vi "ROI entry-ROI text boundary condition.vi"(8 "Error in (no error)":errorcluster, 10 "Image":T1, 11 "XY coordinates in":cluster{"X":i32, "Y":i32}) -> (0 "error out":errorcluster, 3 "XY coordinates out":cluster{"X":i32, "Y":i32})   [LabVIEW 2013]
uses:
  <vilib>/vision/Image Controls.llb/IMAQ Image.ctl
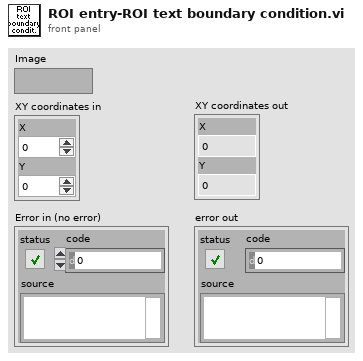
[diagram p1: front panel]
types:
  T1 = typedef "IMAQ Image.ctl" = refnum<image>
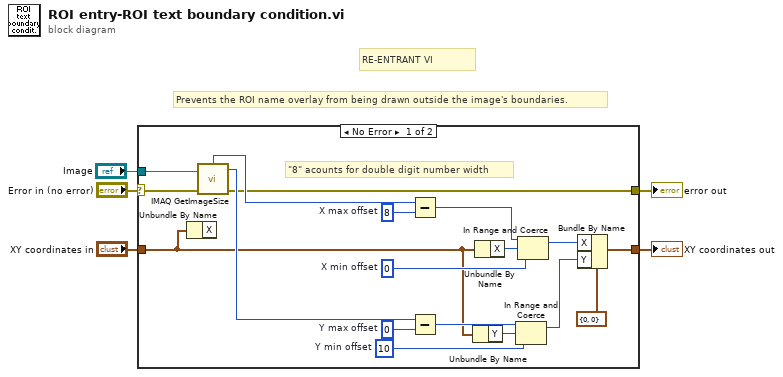
[diagram p0: block diagram]
diagram:
  # "Prevents the ROI name overlay from being drawn outside the image's boundaries."
  # "RE-ENTRANT VI"
  n1 = case shown="No Error" "Error in (no error)" {
    selector: "Error in (no error)" -> [w7 w25]
    tunnel: "XY coordinates in" -> [w8 w24]
    tunnel: [w14 w24] -> w4
    tunnel: [w13 w25] -> w3
    tunnel: "Image" -> [w6 _]
    frame No Error {
      w9 = 10  # Y min offset
      w10 = 0  # X min offset
      w11 = 0  # Y max offset
      w12 = 8  # X max offset
      # "\"8\" acounts for double digit number width"
      n2 = Unbundle By Name(w8) -> ()  [unwired: 1 out]
      n3 = call "IMAQ GetImageSize"("Image"=w6, "error in (no error)"=w7) -> ("Y Resolution"=w19:i32, "X Resolution"=w21:i32, "error out"=w13:errorcluster)  [unwired: 2 in]
      n4 = Subtract(x=w21, y=w12) -> (x-y=w22:i32)
      n5 = Subtract(x=w19, y=w11) -> (x-y=w18:i32)
      n6 = Unbundle By Name(w8) -> ("Y"=w20:i32)
      n7 = Unbundle By Name(w8) -> ("X"=w23:i32)
      n8 = In Range and Coerce(upper limit=w18, x=w20, lower limit=w9) -> (coerced(x)=w15:i32)  [unwired: 1 out]
      n9 = In Range and Coerce(upper limit=w22, x=w23, lower limit=w10) -> (coerced(x)=w16:i32)  [unwired: 1 out]
      n10 = Bundle By Name(cluster=cluster{"X":i32, "Y":i32} {"X"=0, "Y"=0} ("XY coordinates out"), "X"=w16, "Y"=w15) -> (w14:cluster{"X":i32, "Y":i32})
    }
    frame Error {
    }
  }
  "XY coordinates out" <- w4
  "error out" <- w3
